vi "main_MDI.vi"() -> ()   [LabVIEW 2009]
uses:
  FG states.ctl
  MDI_global.vi
  <vilib>/Utility/miscctls.llb/LVBoundsTypeDef.ctl
  <vilib>/Utility/miscctls.llb/LVRectTypeDef.ctl
panel:
  in  "Close app":bool
  in  "window list":u16(ring)
  in  "Remove child window":bool
  in  "Create Child window":bool
  in  "-dummy":bool
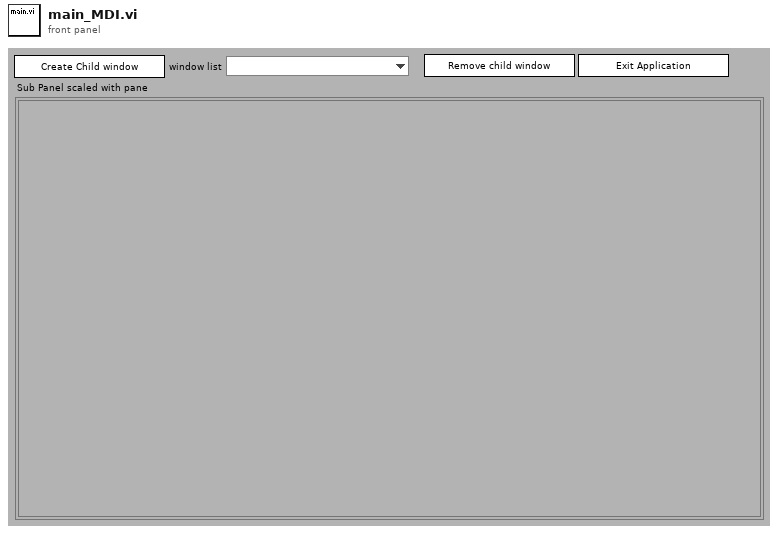
[diagram p1: front panel]
types:
  T1 = typedef "FG states.ctl" = enum16{"init", "add", "replace", "remove", "read"}
  T2 = typedef "LVBoundsTypeDef.ctl" = cluster{"Width":u32, "Height":u32}
  T3 = typedef "LVRectTypeDef.ctl" = cluster{"Left":i16, "Top":i16, "Right":i16, "Bottom":i16}
  T4 = enum32{"Invalid", "Standard", "Closed", "Hidden", "Minimized", "Maximized"}
  T5 = typedef "LVPositionTypeDef.ctl" = cluster{"Left":i32, "Top":i32}
  T6 = typedef "child window props.ctl" = cluster{"WindowTitle":string, "hWnd":u32, "VI Refnum":refnum<vi>}
  T7 = cluster{"Vi tiltle":string, "hWnd":u32, "vi reference out (dup)":refnum<vi>}
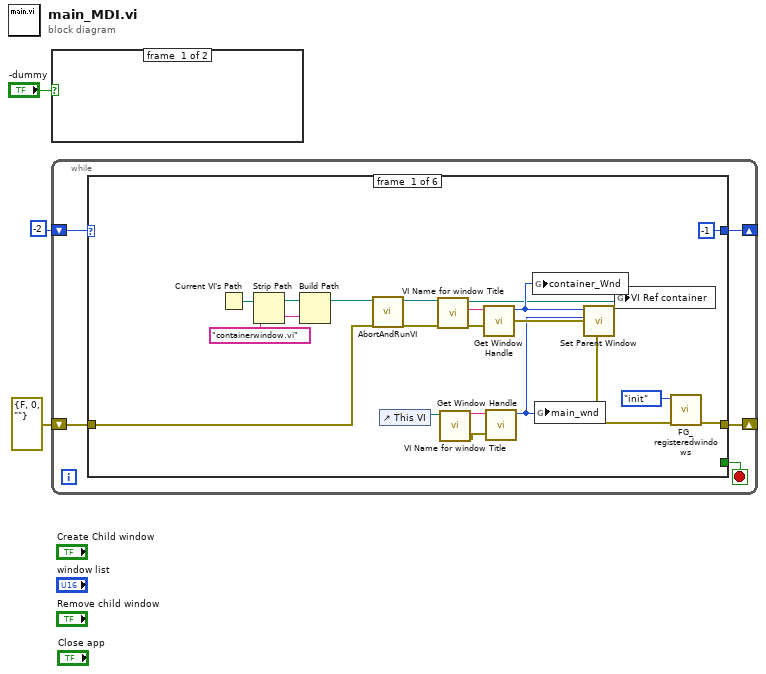
[diagram p0: block diagram]
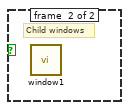
[diagram p2: hidden frame]
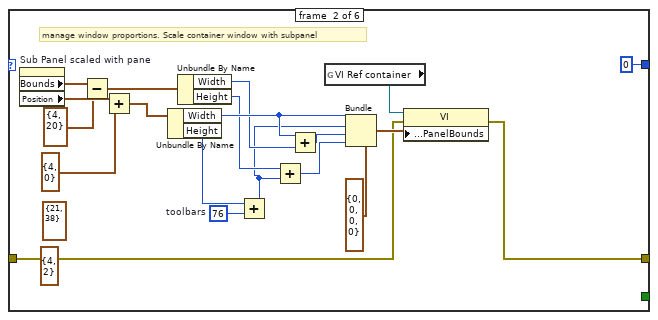
[diagram p3: hidden frame]
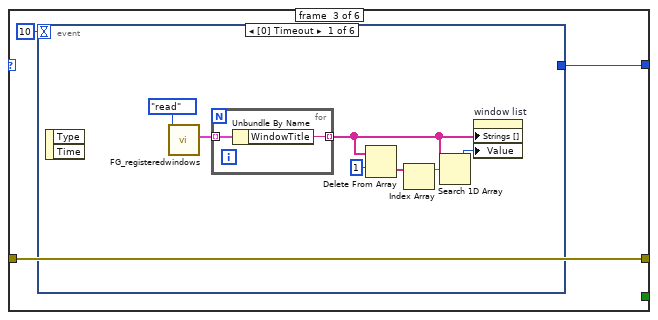
[diagram p4: hidden frame]
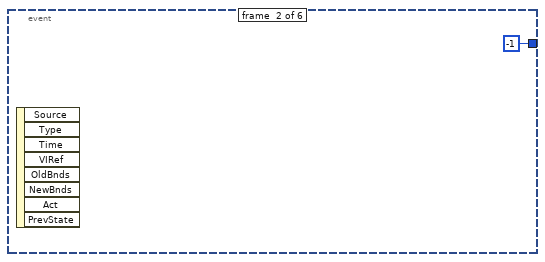
[diagram p5: hidden frame]
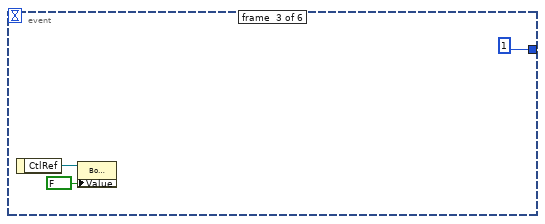
[diagram p6: hidden frame]
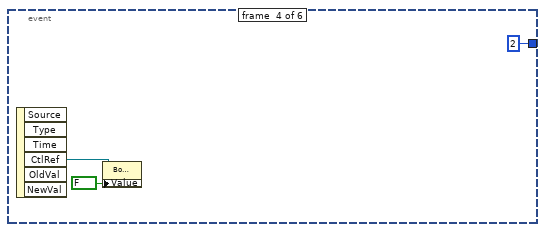
[diagram p7: hidden frame]
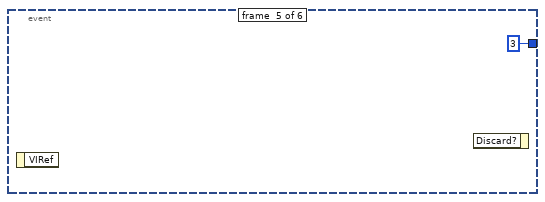
[diagram p8: hidden frame]
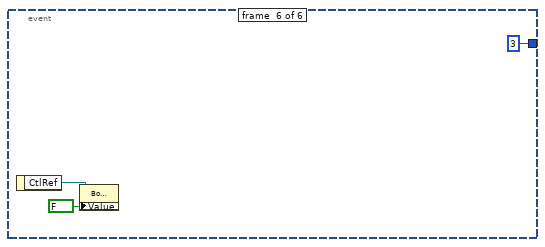
[diagram p9: hidden frame]
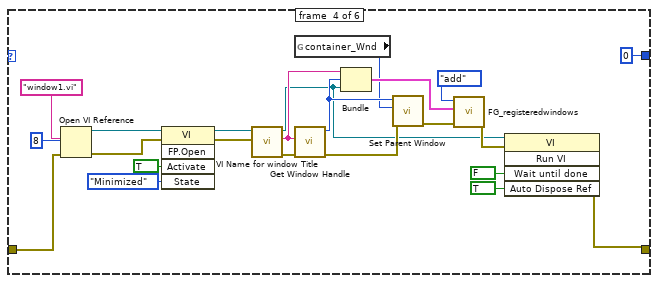
[diagram p10: hidden frame]
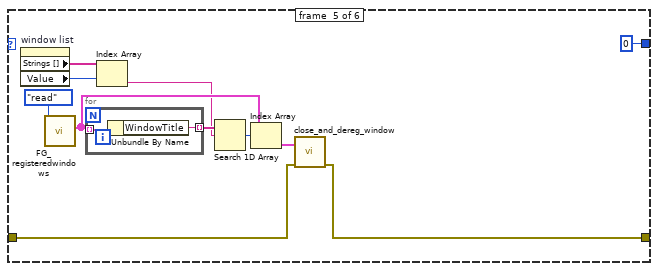
[diagram p11: hidden frame]
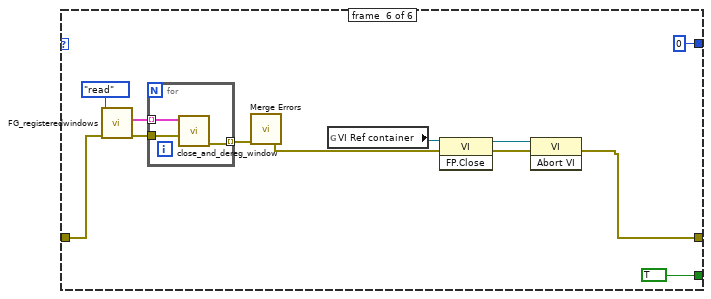
[diagram p12: hidden frame]
diagram:
  n1 = case shown="True" "-dummy" {
    frame #0 {
    }
    frame #1 {
      # "Child windows"
      n2 = call "window1.vi"() -> ()  [unwired: 1 out]
    }
  }
  n3 = while {
    shift-right: [w5] -> _
    shift-left: -2 -> [w8]
    shift-right: [w6] -> _
    shift-left: errorcluster {"status"=FALSE, "code"=0, "source"=""} ("error out") -> [w7]
    stop <- w4 stop-if-true
    n4 = case shown="0, Default" w8 {
      tunnel: w7 -> [w12 w39 w49 w86 w104 w111]
      tunnel: [w23 w38 w49 w76 w97 w107] -> w6
      tunnel: [-1 0 w50 0 0 0] -> w5
      tunnel: [_ _ _ _ _ TRUE] -> w4
      frame #0 {
        n5 = Current VI's Path() -> (path=w25:path)
        n6 = Strip Path(path=w25) -> (stripped path=w24:path)  [unwired: 1 out]
        n7 = Build Path(base path=w24, name or relative path="containerwindow.vi" ("vi path")) -> (appended path=w11:path)
        n8 = call "AbortAndRunVI.vi"("error out"=w12, "appended path"=w11) -> ("error out 4"=w9:errorcluster, "vi reference 4"=w10:refnum<vi>)  [unwired: 8 out]
        n9 = control-ref of="This VI"() -> (w22:refnum<vi>)
        n10 = call "VI Name for window Title.vi"("error in"=w9, "vi reference"=w10) -> ("error out"=w14:errorcluster, "Vi tiltle"=w19:string, "vi reference out (dup)"=w15:refnum<vi>)  [unwired: 7 out]
        n11 = call "VI Name for window Title.vi"("vi reference"=w22) -> ("error out"=w13:errorcluster, "Vi tiltle"=w21:string)  [unwired: 1 in, 8 out]
        n12 = call "Get Window Handle.vi"("error in (no error)"=w14, "window name (\"\")"=w19) -> ("error out"=w18:errorcluster, "hWnd"=w16:u32)  [unwired: 1 in, 3 out]
        n13 = call "Get Window Handle.vi"("error in (no error)"=w13, "window name (\"\")"=w21) -> ("hWnd"=w17:u32)  [unwired: 1 in, 4 out]
        n14 = global write "MDI_global.vi" "container_Wnd"(w16) -> ()
        n15 = global write "MDI_global.vi" "main_wnd"(w17) -> ()
        n16 = call "Set Parent Window.vi"("new parent"=w17, "child"=w16) -> ()  [unwired: 2 in, 8 out]
        n17 = global write "MDI_global.vi" "VI Ref container"(w15) -> ()
        n18 = call "FG_registeredwindows.vi"("error in (no error)"=w18, "action"=FG_states."init") -> ("error out"=w23:errorcluster)  [unwired: 1 in, 8 out]
      }
      frame #1 {
        (unwired) T2 {"Width"=4, "Height"=2} ("y")
        (unwired) T2 {"Width"=21, "Height"=38} ("y")
        w36 = u32 76  # toolbars
        # "manage window proportions. Scale container window with subpanel"
        n19 = property on="Sub Panel scaled with pane" class="SubPnl"() -> ("Bounds"=w33:T2, "Position"=w31:T5)  [unwired: 2 in, 2 out]
        n20 = Subtract(x=w33, y=T2 {"Width"=4, "Height"=20}) -> (x-y=w32:T2)
        n21 = Add(x=w31, y=T2 {"Width"=4, "Height"=0}) -> (x+y=w30:T2)
        n22 = Unbundle By Name(w30) -> ("Width"=w46:u32, "Height"=w35:u32)
        n23 = Unbundle By Name(w32) -> ("Width"=w45:u32, "Height"=w44:u32)
        n24 = Add(x=w35, y=w36) -> (x+y=w34:u32)
        n25 = Add(x=w44, y=w34) -> (x+y=w37:u32)
        n26 = Add(x=w46, y=w45) -> (x+y=w43:u32)
        n27 = global read "MDI_global.vi" "VI Ref container"() -> (w41:refnum<vi>)
        n28 = Bundle(cluster=T3 {"Left"=0, "Top"=0, "Right"=0, "Bottom"=0} ("Front Panel Window:Panel Bounds"), "Left"=w46, "Top"=w34, "Right"=w43, "Bottom"=w37) -> (w42:T3)
        n29 = property class="VI"(reference=w41, error in=w39, "Front Panel.PanelBounds"=w42) -> (error out=w38:errorcluster)  [unwired: 1 out]
      }
      frame #2 {
        n30 = event shown="[0] Timeout" {
          selector: _ -> [_ _ _ _ _ _]
          dyn-events: _ -> [_ _ _ _ _ _]
          timeout: 10 -> [_ _ _ _ _ _]
          tunnel: [_ -1 1 2 3 3] -> w50
          event #0 {
            n31 = event-data() -> ()  [unwired: 3 out]
            n32 = call "FG_registeredwindows.vi"("action"=FG_states."read") -> ("windows"=w56:T6[])  [unwired: 2 in, 8 out]
            n33 = for {
              tunnel: w56 -> [w59] mode=indexing
              tunnel: [w58] -> w53 mode=indexing
              n34 = Unbundle By Name(w59) -> ("WindowTitle"=w58:string)
            }
            n35 = Delete From Array(array=w53, length=1) -> (deleted portion=w54:string[])  [unwired: 1 in, 1 out]
            n36 = Index Array(array=w54) -> (element=w52:string)  [unwired: 1 in]
            n37 = Search 1D Array(1D array=w53, element=w52) -> (index of element=w51:i32)  [unwired: 1 in]
            n38 = property on="window list" class="Ring (strict)"("Strings []"=w53, "Value"=w51) -> ()  [unwired: 2 in, 2 out]
          }
          event #1 {
            n39 = event-data() -> ()  [unwired: 9 out]
          }
          event #2 {
            n40 = event-data() -> ("CtlRef"=w62:refnum<vi>)  [unwired: 1 out]
            n41 = property class="Bool (strict)"(reference=w62, "Value"=FALSE) -> ()  [unwired: 1 in, 2 out]
          }
          event #3 {
            n42 = event-data() -> ("CtlRef"=w64:refnum<vi>)  [unwired: 6 out]
            n43 = property class="Bool (strict)"(reference=w64, "Value"=FALSE) -> ()  [unwired: 1 in, 2 out]
          }
          event #4 {
            n44 = event-data() -> ()  [unwired: 2 out]
            n45 = event-data() -> ()  [unwired: 1 in, 2 out]
          }
          event #5 {
            n46 = event-data() -> ("CtlRef"=w68:refnum<vi>)  [unwired: 1 out]
            n47 = property class="Bool (strict)"(reference=w68, "Value"=FALSE) -> ()  [unwired: 1 in, 2 out]
          }
        }
      }
      frame #3 {
        n48 = Open VI Reference(vi path="window1.vi", options=8, error in (no error)=w86) -> (vi reference=w81:refnum<vi>, error out=w80:errorcluster)  [unwired: 3 out]
        n49 = invoke class="VI" method="FP.Open"(reference=w81, error in=w80, "Activate"=TRUE ("Activate?"), "State"=T4."Minimized") -> (reference out=w79:refnum<vi>, error out=w78:errorcluster)  [unwired: 1 in, 3 out]
        n50 = call "VI Name for window Title.vi"("error in"=w78, "vi reference"=w79) -> ("error out"=w85:errorcluster, "Vi tiltle"=w83:string, "vi reference out (dup)"=w73:refnum<vi>)  [unwired: 7 out]
        n51 = global read "MDI_global.vi" "container_Wnd"() -> (w82:u32)
        n52 = call "Get Window Handle.vi"("error in (no error)"=w85, "window name (\"\")"=w83) -> ("error out"=w84:errorcluster, "hWnd"=w91:u32)  [unwired: 1 in, 3 out]
        n53 = Bundle("Vi tiltle"=w83, "hWnd"=w91, "vi reference out (dup)"=w73) -> (w89:T7)  [unwired: 1 out]
        n54 = call "Set Parent Window.vi"("error in (no error)"=w84, "new parent"=w82, "child"=w91) -> ("error out"=w88:errorcluster)  [unwired: 1 in, 7 out]
        n55 = call "FG_registeredwindows.vi"("error in (no error)"=w88, "window"=w89, "action"=FG_states."add") -> ("error out"=w77:errorcluster)  [unwired: 8 out]
        n56 = invoke class="VI" method="Run VI"(reference=w73, error in=w77, "Wait until done"=FALSE ("Wait Until Done"), "Auto Dispose Ref"=TRUE ("Auto Dispose Reference")) -> (error out=w76:errorcluster)  [unwired: 1 in, 4 out]
      }
      frame #4 {
        n57 = property on="window list" class="Ring (strict)"() -> ("Strings []"=w96:string[], "Value"=w95:u16)  [unwired: 2 in, 2 out]
        n58 = call "FG_registeredwindows.vi"("action"=FG_states."read") -> ("windows"=w100:T6[])  [unwired: 2 in, 8 out]
        n59 = for {
          tunnel: w100 -> [w106] mode=indexing
          tunnel: [w105] -> w101 mode=indexing
          n60 = Unbundle By Name(w106) -> ("WindowTitle"=w105:string)
        }
        n61 = Index Array(array=w96, index=w95) -> (element=w94:string)
        n62 = Search 1D Array(1D array=w101, element=w94) -> (index of element=w99:i32)  [unwired: 1 out]
        n63 = Index Array(array=w100, index=w99) -> (element=w98:T6)
        n64 = call "close_and_dereg_window.vi"("error in"=w104, "window"=w98) -> ("error out"=w97:errorcluster)  [unwired: 8 out]
      }
      frame #5 {
        n65 = call "FG_registeredwindows.vi"("error in (no error)"=w111, "action"=FG_states."read") -> ("error out"=w113:errorcluster, "windows"=w114:T6[])  [unwired: 1 in, 7 out]
        n66 = for {
          tunnel: w114 -> [w121] mode=indexing
          tunnel: w113 -> [w120]
          tunnel: [w119] -> w112 mode=indexing
          n67 = call "close_and_dereg_window.vi"("error in"=w120, "window"=w121) -> ("error out"=w119:errorcluster)  [unwired: 8 out]
        }
        n68 = call <vilib>:"Merge Errors.vi"("error array in"=w112) -> ("error out"=w110:errorcluster)  [unwired: 3 in, 3 out]
        n69 = global read "MDI_global.vi" "VI Ref container"() -> (w116:refnum<vi>)
        n70 = invoke class="VI" method="FP.Close"(reference=w116, error in=w110) -> (reference out=w109:refnum<vi>, error out=w108:errorcluster)  [unwired: 1 in, 1 out]
        n71 = invoke class="VI" method="Abort VI"(reference=w109, error in=w108) -> (error out=w107:errorcluster)  [unwired: 1 in, 2 out]
      }
    }
  }
